vi "Actor Core.vi"(8 "error in":errorcluster, 11 "Single Assert Display in":refnum<class "Single Assert Display.lvclass">) -> (0 "error out":errorcluster, 3 "Actor out":refnum<class "Actor.lvclass">)   [LabVIEW 2016, in "Assert API Components.lvlib" / "Assert Display.lvlib" / "Single Assert Display.lvlib" / "Single Assert Display.lvclass"]
doc: "(<B>Filename</B>: Actor Framework.lvlib:Actor.lvclass:Actor Core.vi)\n\nReceives messages to the actor, reacts to them, and initiates any error handling that may shut the actor down.\n\nDescendant classes may override this VI to append parallel tasks for the actor to complete while it handles messages. Overrides use the Call Parent Method node."
uses:
  Single Assert Display.lvclass
  C:/Program Files (x86)/National Instruments/LabVIEW 2016/vi.lib/ActorFramework/Actor/Actor.lvclass
  D:/Work/Projects/Actor_Assert_API/Base UI Actor/Base UI Actor/Base UI Actor.lvclass
  <vilib>/ActorFramework/Actor/Actor.lvclass
  Assert API Components/Message Data.ctl
  Assert API Components/VI References.ctl
  Base UI Actor/Base UI Actor/Base UI Actor.lvclass/Base UI Actor.ctl
  <vilib>/ActorFramework/Actor/Actor.lvclass/Actor.ctl
  <vilib>/ActorFramework/Message Enqueuer/Message Enqueuer.lvclass/Message Enqueuer.ctl
  Single Assert Display.lvclass/Single Assert Display.ctl
  <vilib>/ActorFramework/Message Enqueuer/Init from Existing Queue.vi
  <vilib>/ActorFramework/Message Enqueuer/Enqueue.vi
  <vilib>/ActorFramework/Stop Msg/Stop Msg.lvclass
  C:/Program Files (x86)/National Instruments/LabVIEW 2016/vi.lib/ActorFramework/Message/Message.lvclass
  <vilib>/ActorFramework/Message Priority Queue/Priority Enqueue.vi
  Base UI Actor/Base UI Actor/Base UI Actor.lvclass
  <vilib>/ActorFramework/Message Enqueuer/Message Enqueuer.lvclass
  Assert API Components/Assert API Components.lvlib
panel:
  out "Assert Message":T1
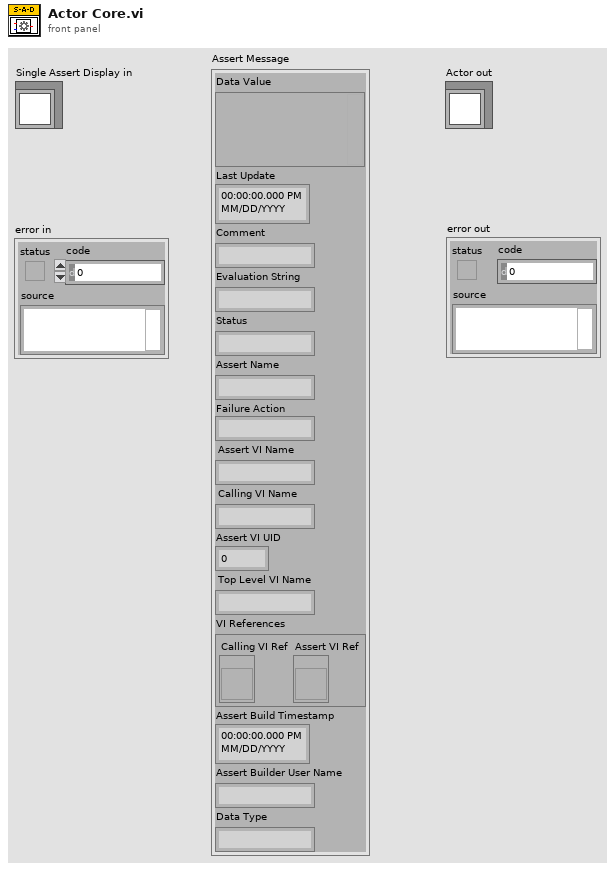
[diagram p1: front panel]
types:
  T1 = typedef "Assert API Components.lvlib/Message Data.ctl" = cluster{"Data Value":variant, "Last Update":timestamp, "Comment":string, "Evaluation String":string, "Status":string, "Assert Name":string, "Failure Action":string, "Assert VI Name":string, "Calling VI Name":string, "Assert VI UID":i32, "Top Level VI Name":string, "VI References":T2, "Assert Build Timestamp":timestamp, "Assert Builder User Name":string, "Data Type":string}
  T2 = typedef "Assert API Components.lvlib/VI References.ctl" = cluster{"Calling VI Ref":refnum<vi>, "Assert VI Ref":refnum<vi>}
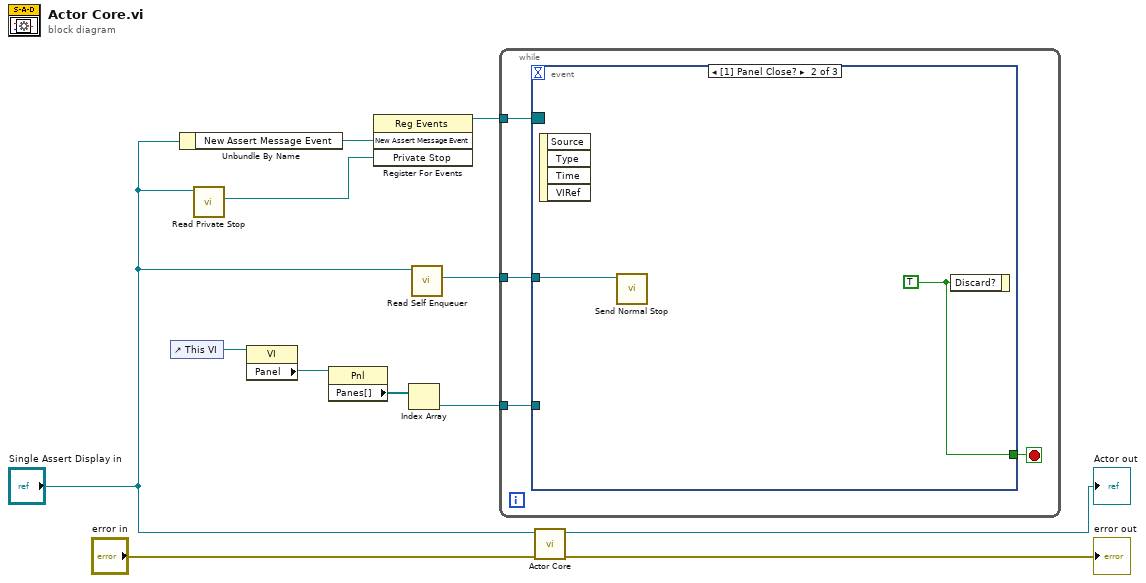
[diagram p0: block diagram]
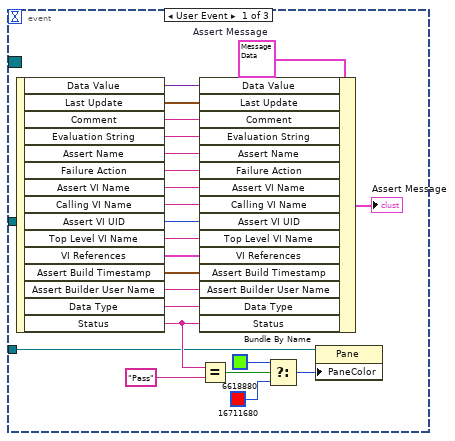
[diagram p2: hidden frame]
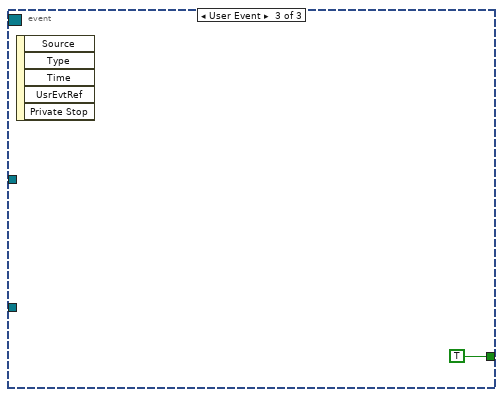
[diagram p3: hidden frame]
diagram:
  n1 = control-ref of="This VI"() -> (w6:refnum<vi>)
  n2 = Unbundle By Name("Single Assert Display in") -> ("New Assert Message Event"=w9:refnum<user-event>)
  n3 = call "Read Private Stop.vi"("Base UI Actor in"="Single Assert Display in") -> ("Private Stop"=w8:refnum<user-event>)  [unwired: 10 in]
  n4 = property class="VI"(reference=w6) -> ("Panel"=w5:refnum<vi>)  [unwired: 1 in, 2 out]
  n5 = property class="Pnl"(reference=w5) -> ("Panes[]"=w4:refnum<vi>[])  [unwired: 1 in, 2 out]
  n6 = register-events(w9, w8) -> (reference out=w7:refnum<event-registration>)  [unwired: 2 in, 1 out]
  n7 = Index Array(array=w4) -> (element=w3:refnum<vi>)  [unwired: 1 in]
  n8 = call <vilib>:"Read Self Enqueuer.vi"("Actor"="Single Assert Display in") -> ("Self Enqueuer"=w1:refnum<class "Message Enqueuer.lvclass">)  [unwired: 10 in]
  n9 = while {
    tunnel: w7 -> [w16]
    tunnel: w3 -> [w14]
    tunnel: w1 -> [w13]
    stop <- w15 stop-if-true
    n10 = event shown="[1] Panel Close?" {
      selector: w16 -> [_ _ _]
      dyn-events: _ -> [_ _ _]
      timeout: _ -> [_ _ _]
      tunnel: [_ w41 TRUE] -> w15
      tunnel: w14 -> [w17 _ _]
      tunnel: w13 -> [_ w40 _]
      event User Event {
        w39 = T1 {"Data Value"=variant, "Last Update"=timestamp(0 s since 1904-01-01), "Comment"="", "Evaluation String"="", "Status"="", "Assert Name"="", "Failure Action"="", "Assert VI Name"="", "Calling VI Name"="", "Assert VI UID"=0, "Top Level VI Name"="", "VI References"={"Calling VI Ref"=refnum, "Assert VI Ref"=refnum}, "Assert Build Timestamp"=timestamp(0 s since 1904-01-01), "Assert Builder User Name"="", "Data Type"=""}  # Assert Message
        n11 = event-data() -> ("Data Value"=w38:variant, "Last Update"=w37:timestamp, "Comment"=w36:string, "Evaluation String"=w35:string, "Assert Name"=w34:string, "Failure Action"=w33:string, "Assert VI Name"=w32:string, "Calling VI Name"=w31:string, "Assert VI UID"=w30:i32, "Top Level VI Name"=w29:string, "VI References"=w28:T2, "Assert Build Timestamp"=w27:timestamp, "Assert Builder User Name"=w26:string, "Data Type"=w25:string, "Status"=w23:string)  [unwired: 1 in]
        n12 = Bundle By Name(cluster=w39, "Data Value"=w38, "Last Update"=w37, "Comment"=w36, "Evaluation String"=w35, "Assert Name"=w34, "Failure Action"=w33, "Assert VI Name"=w32, "Calling VI Name"=w31, "Assert VI UID"=w30, "Top Level VI Name"=w29, "VI References"=w28, "Assert Build Timestamp"=w27, "Assert Builder User Name"=w26, "Data Type"=w25, "Status"=w23) -> (→"Assert Message":T1)
        n13 = Equal?(x=w23, y="Pass") -> (x = y?=w21:bool)
        n14 = Select(t=u32 6618880, s=w21, f=u32 16711680) -> (s? t:f=w18:u32)
        n15 = property class="Pane"(reference=w17, "PaneColor"=w18) -> ()  [unwired: 1 in, 2 out]
      }
      event Panel Close? {
        w41 = TRUE ("Discard?")
        n16 = event-data() -> ()  [unwired: 1 in, 4 out]
        n17 = call <vilib>:"Send Normal Stop.vi"("Message Enqueuer"=w40) -> ()  [unwired: 10 in, 1 out]
        n18 = event-data("Discard?"=w41) -> ()  [unwired: 1 in, 1 out]
      }
      event User Event {
        n19 = event-data() -> ()  [unwired: 1 in, 5 out]
      }
    }
  }
  n20 = call-parent "Actor Core.vi"("error in"="error in", "Actor in"="Single Assert Display in") -> ("error out"=→"error out":errorcluster, "Actor out"=→"Actor out":refnum<class "Actor.lvclass">)  [unwired: 8 in]
